vi "ConnectHardware.vi"(8 "Error In":errorcluster, 11 "MainData":T1) -> (0 "Error Out":errorcluster, 3 "MainData out":T1)   [LabVIEW 2019, in "MainController.lvlib"]
uses:
  MainController.lvlib
  Cluster - MainData.ctl
  All Message Queues.ctl
  Cluster - MainControllerMessage.ctl
  Enum - MainState.ctl
  AutoMode/Cluster - AutoModeMessage.ctl
  AutoMode/Enum - AutoModeState.ctl
  ManualMode/Cluster - ManualModeMessageCluster.ctl
  ManualMode/Enum - ManualModeMessage.ctl
  Settings/CTL_MessageCluster.ctl
  Settings/CTL_SettingsMessage.ctl
  EventLogger/Cluster - MessageCluster.ctl
  EventLogger/Enum - Message.ctl
  Cluster - HardwareConfiguration.ctl
  Cluster - LoggingConfiguration.ctl
  Cluster - TestSettings.ctl
  UI State.ctl
  UI Data.ctl
  Mark10 API/Cluster - COMSettings.ctl
  Mark10 API/Enum - TravelUnit.ctl
  Mark10 API/WriteTravelUnits.vi
  Mark10 API/Mark 10 TSTM-DC.lvlib
  EventLogger/EventLogger.lvlib
  AutoMode/AutoMode.lvlib
  ManualMode/ManualMode.lvlib
  Settings/Settings.lvlib
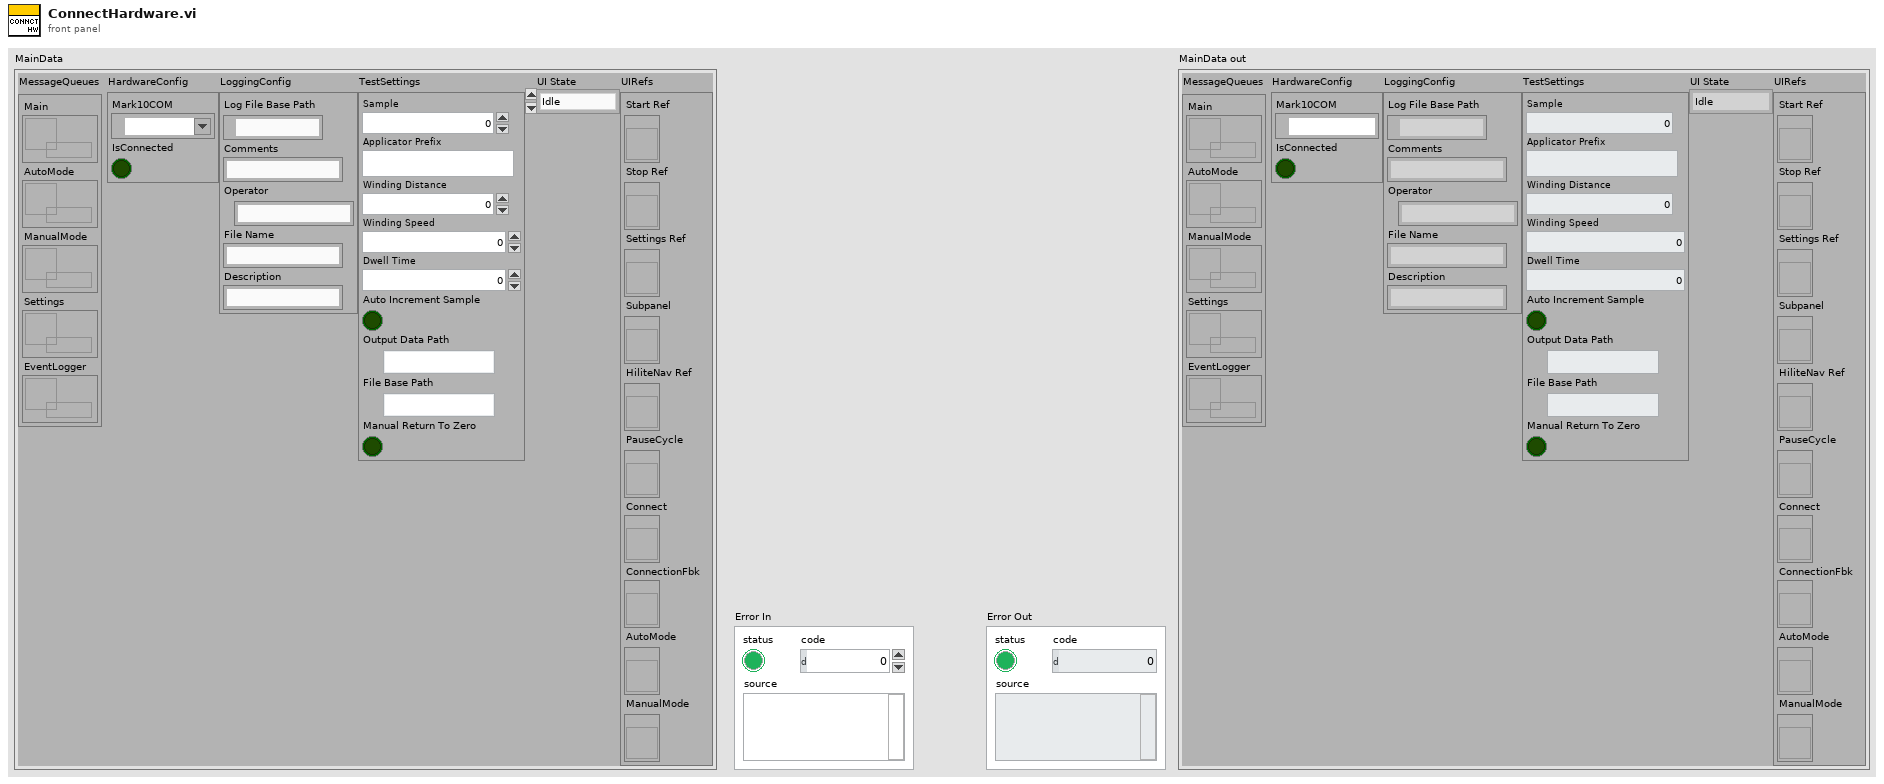
[diagram p1: front panel]
types:
  T1 = typedef "MainController.lvlib/Cluster - MainData.ctl" = cluster{"MessageQueues":T2, "HardwareConfig":T3, "LoggingConfig":T4, "TestSettings":T5, "UI State":T6, "UIRefs":T7}
  T2 = typedef "MainController.lvlib/All Message Queues.ctl" = cluster{"Main":refnum<queue>, "AutoMode":refnum<queue>, "ManualMode":refnum<queue>, "Settings":refnum<queue>, "EventLogger":refnum<queue>}
  T3 = typedef "MainController.lvlib/Cluster - HardwareConfiguration.ctl" = cluster{"Mark10COM":refnum<visa-resource-name>, "IsConnected":bool}
  T4 = typedef "MainController.lvlib/Cluster - LoggingConfiguration.ctl" = cluster{"Log File Base Path":path, "Comments ":string, "Operator":string, "File Name":string, "Description":string}
  T5 = typedef "MainController.lvlib/Cluster - TestSettings.ctl" = cluster{"Sample":u32, "Applicator Prefix":string, "Winding Distance":dbl, "Winding Speed":dbl, "Dwell Time":dbl, "Auto Increment Sample":bool, "Output Data Path":path, "File Base Path":path, "Manual Return To Zero":bool}
  T6 = typedef "MainController.lvlib/UI State.ctl" = enum16{"Idle", "AutoIdle", "AutoRunning", "ManualMode", "Settings"}
  T7 = typedef "MainController.lvlib/UI Data.ctl" = cluster{"Start Ref":refnum<vi>, "Stop Ref":refnum<vi>, "Settings Ref":refnum<vi>, "Subpanel":refnum<vi>, "HiliteNav Ref":refnum<vi>, "PauseCycle":refnum<vi>, "Connect":refnum<vi>, "ConnectionFbk":refnum<vi>, "AutoMode":refnum<vi>, "ManualMode":refnum<vi>}
  T8 = typedef "MainController.lvlib/Enum - MainState.ctl" = enum16{"Initialize", "InitUIRefs", "LaunchSettings", "LaunchAutoMode", "LaunchManualMode", "LaunchTestReport", "ConnectHardware", "DisconnectHardware", "HiliteNavItems", "StartAutoMode", "PauseAutoMode", "StopAutoMode", "ShowFlyout", "HideFlyout", "BroadcastSettings", "PickupTestSettings", "BroadcastHW", "AutoTestDone", "DAQStatus", "UpdateCommandBar", "Error", "RecieveError", "Exit"}
  T9 = typedef "Mark 10 TSTM-DC.lvlib/Enum - TravelUnit.ctl" = enum16{"Revolutions", "Degrees"}
  T10 = typedef "Mark 10 TSTM-DC.lvlib/Cluster - COMSettings.ctl" = cluster{"baud rate":u32, "data bits":u16, "parity":enum16{"None", "Odd", "Even", "Mark", "Space"}, "stop bits":u16, "flow control":u16}
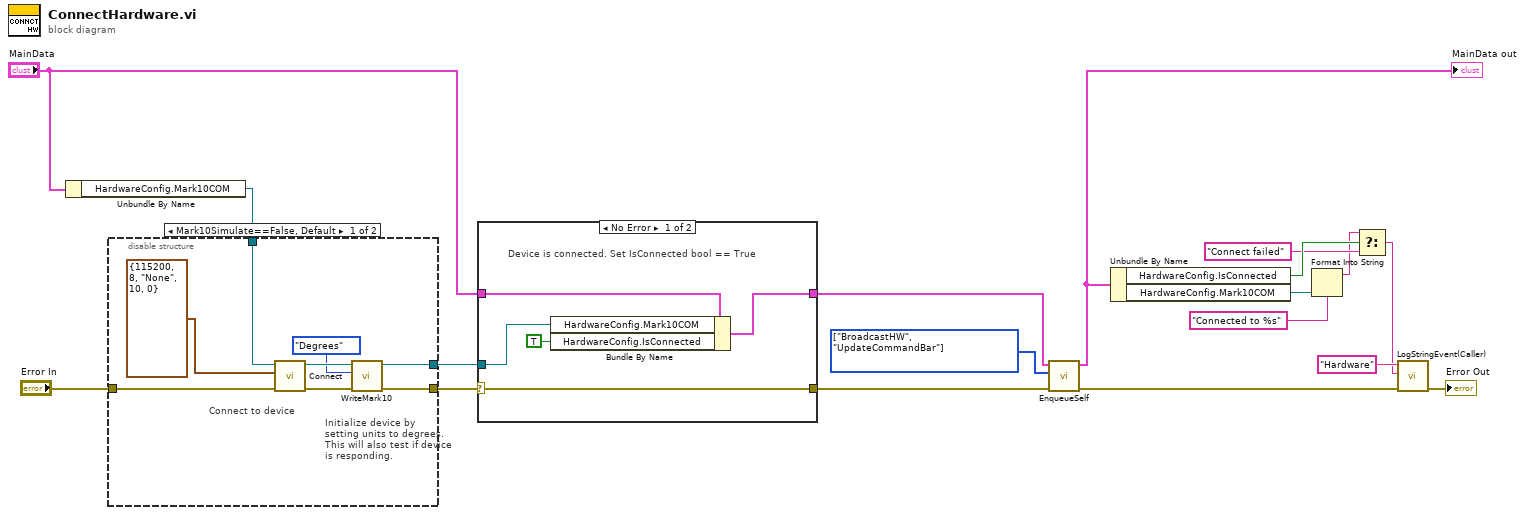
[diagram p0: block diagram]
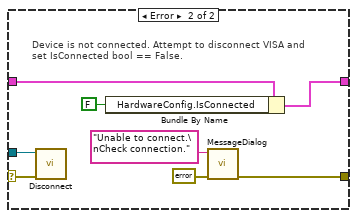
[diagram p3: hidden frame]
diagram:
  w16 = T8[] [enum."BroadcastHW", enum."UpdateCommandBar"] items=["Initialize", "InitUIRefs", "LaunchSettings", "LaunchAutoMode", "LaunchManualMode", "LaunchTestReport", "ConnectHardware", "DisconnectHardware", "HiliteNavItems", "StartAutoMode", "PauseAutoMode", "StopAutoMode", "ShowFlyout", "HideFlyout", "BroadcastSettings", "PickupTestSettings", "BroadcastHW", "AutoTestDone", "DAQStatus", "UpdateCommandBar", "Error", "RecieveError", "Exit"] ("Message")
  n1 = Unbundle By Name("MainData") -> ("HardwareConfig.Mark10COM"=w12:refnum<visa-resource-name>)
  n2 = disable-structure shown="Mark10Simulate==False, Default" {
    disable-tunnel: [w23 w27] -> w18
    disable-tunnel: [w22 w28] -> w10
    disable-tunnel: "Error In" -> [w20 w28]
    disable-tunnel: w12 -> [w19 w27]
    frame condition #0 (active) {
      # "Initialize device by\nsetting units to degrees.\nThis will also test if device\nis responding."
      # "Connect to device"
      n3 = call "Connect.vi"("error in (no error)"=w20, "COM Settings"=T10 {"baud rate"=115200, "data bits"=8, "parity"=enum."None", "stop bits"=10, "flow control"=0}, "VISA resource name"=w19) -> ("error out"=w24:errorcluster, "VISA resource name out"=w25:refnum<visa-resource-name>)  [unwired: 7 in]
      n4 = call-poly "WriteMark10.vi"("error in"=w24, "TravelUnit"=Enum_-_TravelUnit."Degrees", "VISA resource name"=w25) -> ("error out"=w22:errorcluster, "VISA resource name out"=w23:refnum<visa-resource-name>)  [unwired: 7 in]
    }
    frame condition #1 {
    }
  }
  n5 = case shown="No Error" w10 {
    selector: w10 -> [w32 w35]
    tunnel: w18 -> [w33 w34]
    tunnel: [w32 w36] -> w17
    tunnel: "MainData" -> [w31 w39]
    tunnel: [w30 w40] -> w11
    frame No Error {
      # "Device is connected. Set IsConnected bool == True"
      n6 = Bundle By Name(cluster=w31, "HardwareConfig.Mark10COM"=w33, "HardwareConfig.IsConnected"=TRUE) -> (w30:T1)
    }
    frame Error {
      # "Device is not connected. Attempt to disconnect VISA and\nset IsConnected bool == False."
      n7 = call "Disconnect.vi"("error in (no error)"=w35, "VISA resource name"=w34) -> ()  [unwired: 8 in, 2 out]
      n8 = Bundle By Name(cluster=w39, "HardwareConfig.IsConnected"=FALSE) -> (w40:T1)
      n9 = call "MessageDialog.vi"("error in (no error)"=errorcluster {"status"=FALSE, "code"=0, "source"=""} ("error IO"), "Message"="Unable to connect.\nCheck connection.") -> ("error out"=w36:errorcluster)  [unwired: 9 in]
    }
  }
  n10 = call "EnqueueSelf.vi"("Error In"=w17, "Messages"=w16, "MainData"=w11) -> ("Error Out"=w14:errorcluster, "MainData out"=w7:T1)  [unwired: 7 in]
  "MainData out" <- w7
  n11 = Unbundle By Name(w7) -> ("HardwareConfig.IsConnected"=w6:bool, "HardwareConfig.Mark10COM"=w3:refnum<visa-resource-name>)
  n12 = Format Into String(format string="Connected to %s", w3) -> (resulting string=w1:string)  [unwired: 2 in, 1 out]
  n13 = Select(t=w1, s=w6, f="Connect failed") -> (s? t:f=w4:string)
  n14 = call "LogStringEvent(Caller).vi"("Error In"=w14, "Data"=w4, "Field"="Hardware") -> ("Error Out"=→"Error Out":errorcluster)  [unwired: 8 in]
